vi "FTW-Actor-Initialized.vi"(0 "FTW Actor Instance":refnum<class "FTW-ActorInstance.lvclass">, 5 "Initialized Response":string, 11 "error in":errorcluster) -> (4 "FTW Actor Instance out":refnum<class "FTW-ActorInstance.lvclass">, 15 "error out":errorcluster)   [LabVIEW 2012, in "FTW-Actor.lvlib" / "FTW-ActorInstance.lvclass"]
uses:
  FTW-ActorInstance.lvclass
  Endpoint/FTW-Endpoint.lvclass
  FTW-ActorInstance.lvclass/FTW-ActorInstance.ctl
panel:
  # "Inputs"
  # "Outputs"
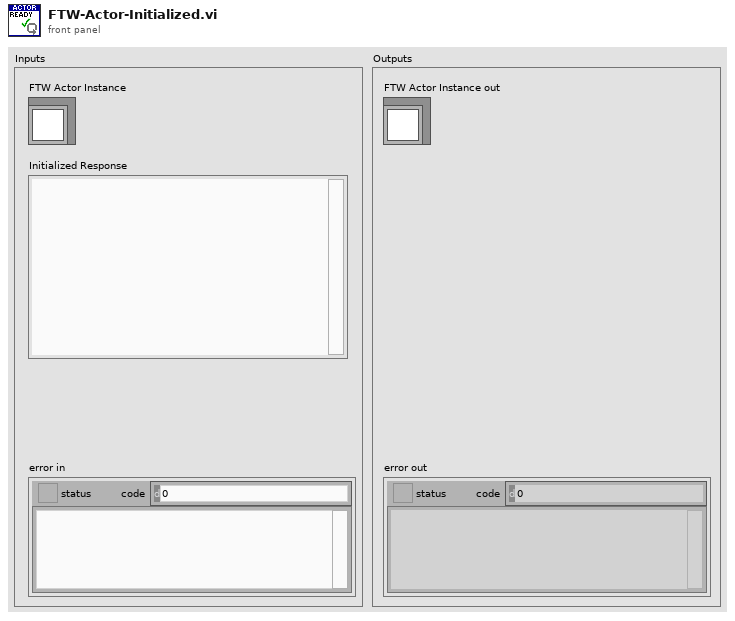
[diagram p1: front panel]
types:
  T1 = enum16{"Instance Initializing", "Instance Initialized", "Instance Job", "Instance Handle Request", "Instance Shutting Down", "Instance Destroyed"}
  T2 = typedef "FTW-Actor.lvlib/FTW-Actor-Address.ctl" = string
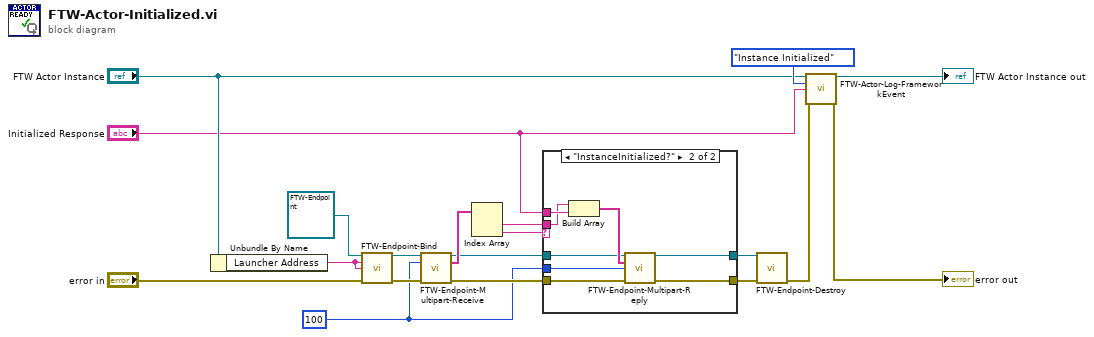
[diagram p0: block diagram]
diagram:
  w1 = 100
  n1 = Unbundle By Name("FTW Actor Instance") -> ("Launcher Address"=w12:T2)
  n2 = call-dynamic "FTW-Endpoint-Bind.vi"("FTW Endpoint"=refnum<class "FTW-Endpoint.lvclass"> refnum, "Endpoint Address"=w12, "Requested Identity"=w12, "error in"="error in") -> ("FTW Endpoint out"=w16:refnum<class "FTW-Endpoint.lvclass">, "error out"=w15:errorcluster)  [unwired: 8 in, 2 out]
  n3 = call-dynamic "FTW-Endpoint-Multipart-Receive.vi"("FTW Endpoint"=w16, "Timeout"=w1, "error in"=w15) -> ("FTW Endpoint out"=w5:refnum<class "FTW-Endpoint.lvclass">, "Message Received"=w10:string[], "error out"=w13:errorcluster)  [unwired: 9 in, 1 out]
  n4 = Index Array(array=w10) -> (element #1=w7:string, element #2=w9:string)  [unwired: 2 in]
  n5 = case shown="\"InstanceInitialized?\"" w9 {
    tunnel: w13 -> [w21 w29]
    tunnel: [w20 w28] -> w8
    tunnel: w7 -> [_ w26]
    tunnel: "Initialized Response" -> [_ w27]
    tunnel: w5 -> [w20 w24]
    tunnel: [w21 w23] -> w4
    tunnel: w1 -> [_ w22]
    frame Default {
    }
    frame "InstanceInitialized?" {
      n6 = Build Array(w26, w27) -> (w25:string[])
      n7 = call-dynamic "FTW-Endpoint-Multipart-Reply.vi"("FTW Endpoint"=w24, "Multipart Message"=w25, "Timeout"=w22, "error in"=w29) -> ("FTW Endpoint out"=w28:refnum<class "FTW-Endpoint.lvclass">, "error out"=w23:errorcluster)  [unwired: 9 in, 1 out]
    }
  }
  n8 = call-dynamic "FTW-Endpoint-Destroy.vi"("FTW Endpoint"=w8, "error in"=w4) -> ("error out"=w3:errorcluster)  [unwired: 13 in]
  n9 = call "FTW-Actor-Log-FrameworkEvent.vi"("FTW Actor Instance"="FTW Actor Instance", "Framework Event"=T1."Instance Initialized", "Event Data"="Initialized Response", "error in"=w3) -> ("FTW Actor Instance out"=→"FTW Actor Instance out":refnum<class "FTW-ActorInstance.lvclass">, "error out"=→"error out":errorcluster)  [unwired: 10 in]
